vi "VMI_calculate_timing.vi"(4 "Peakfind total time":dbl, 5 "Camera_Total_loop time":dbl, 6 "Number of image loops":dbl, 7 "Total loop Number":dbl) -> (1 "AveragePeak find time":dbl, 2 "Average Image Loop time":dbl, 3 "Time per Analysis loop":dbl)   [LabVIEW 2019]
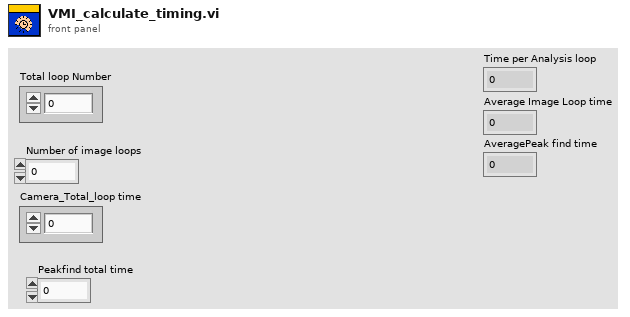
[diagram p1: front panel]
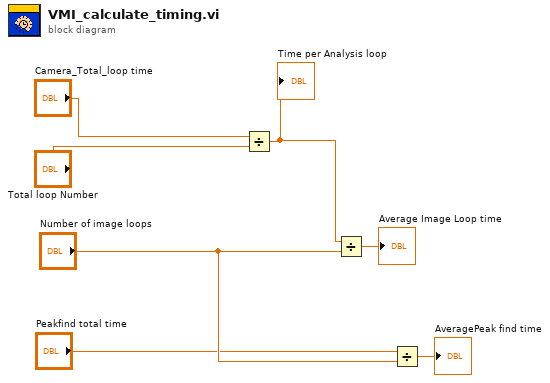
[diagram p0: block diagram]
diagram:
  n1 = Divide(x="Camera_Total_loop time", y="Total loop Number") -> (x/y=w5:dbl)
  "Time per Analysis loop" <- w5
  n2 = Divide(x=w5, y="Number of image loops") -> (x/y=→"Average Image Loop time":dbl)
  n3 = Divide(x="Peakfind total time", y="Number of image loops") -> (x/y=→"AveragePeak find time":dbl)
